vi "Create Mask By Alpha.vi"(10 "Transparency Thresh":u8=127, 11 "image data":T1) -> (3 "masked image data":T1)   [LabVIEW 2011]
uses:
  <vilib>/picture/picture.llb/imagedata.ctl
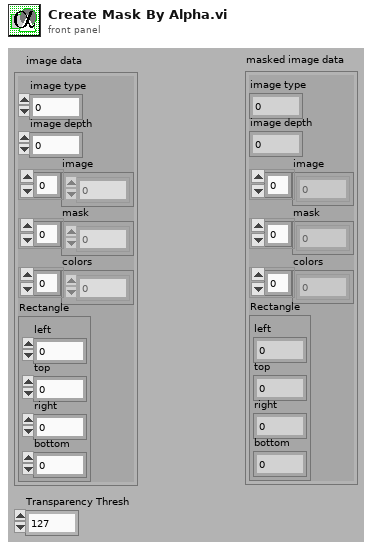
[diagram p1: front panel]
types:
  T1 = typedef "imagedata.ctl" = cluster{"image type":i32, "image depth":i32, "image":u8[], "mask":u8[], "colors":u32[], "Rectangle":cluster{"left":i16, "top":i16, "right":i16, "bottom":i16}}
  T2 = cluster{"left":i16, "top":i16, "right":i16, "bottom":i16}
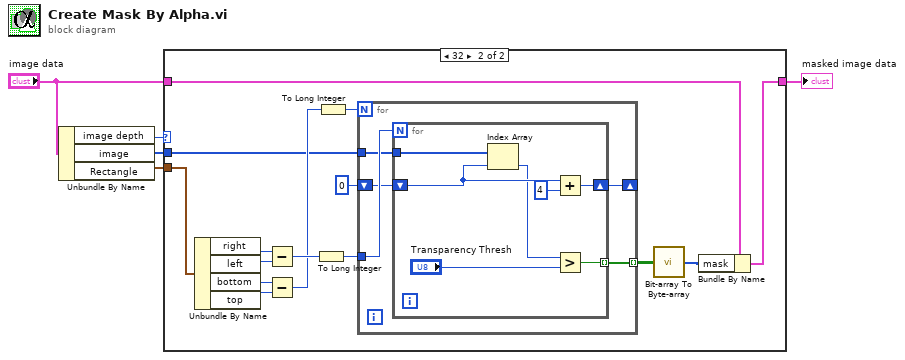
[diagram p0: block diagram]
diagram:
  n1 = Unbundle By Name("image data") -> ("image depth"=w5:i32, "image"=w3:u8[], "Rectangle"=w4:T2)
  n2 = case shown="32" w5 {
    tunnel: w4 -> [_ w21]
    tunnel: w3 -> [_ w14]
    tunnel: "image data" -> [w6 w10]
    tunnel: [w6 w9] -> w1
    frame Default {
    }
    frame 32 {
      n3 = Unbundle By Name(w21) -> ("right"=w20:i16, "left"=w19:i16, "bottom"=w18:i16, "top"=w17:i16)
      n4 = Subtract(x=w20, y=w19) -> (x-y=w16:i16)
      n5 = Subtract(x=w18, y=w17) -> (x-y=w15:i16)
      n6 = To Long Integer(number=w16) -> (32bit integer=w8:i32)
      n7 = To Long Integer(number=w15) -> (32bit integer=w7:i32)
      n8 = for {
        N: w7 -> [_]
        tunnel: w8 -> [w26]
        tunnel: w14 -> [w25]
        shift-right: [w23] -> _
        shift-left: 0 -> [w24]
        tunnel: [w22] -> w12 mode=indexing
        n9 = for {
          N: w26 -> [_]
          tunnel: w25 -> [w33]
          shift-right: [w32] -> w23
          shift-left: w24 -> [w31]
          tunnel: [w27] -> w22 mode=indexing
          n10 = Index Array(array=w33, index=w31) -> (element=w29:u8)
          n11 = Add(x=w31, y=4) -> (x+y=w32:i32)
          n12 = Greater?(x=w29, y="Transparency Thresh") -> (0:w27:bool)
        }
      }
      n13 = call <vilib>:"Bit-array To Byte-array.vi"("bit array"=w12) -> ("byte array"=w11:u8[])
      n14 = Bundle By Name(cluster=w10, "mask"=w11) -> (w9:T1)
    }
  }
  "masked image data" <- w1
